vi "PDE_Cal Coef Mtrx.vi"(8 "length":i32, 9 "ks":dbl, 10 "end type":T1 items=["Dirichlet", "Neumann"], 11 "start type":T1 items=["Dirichlet", "Neumann"]) -> (0 "error":i32, 2 "LU of A":T2, 3 "A":T4)   [LabVIEW 2020, in "NI_PDE.lvlib"]
uses:
  <vilib>/gmath/NI_PDE.lvlib
  <vilib>/gmath/pde.llb/Common/PDE_BC Type.ctl
  <vilib>/Analysis/Matrix/Datatypes/RealMatrix.ctl
  <vilib>/Analysis/NI_AALPro.lvlib
  <vilib>/Analysis/Matrix/NI_Matrix.lvlib
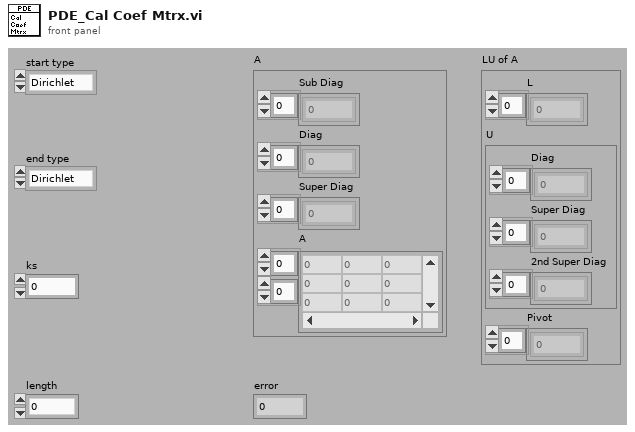
[diagram p1: front panel]
types:
  T1 = typedef "NI_PDE.lvlib/PDE_BC Type.ctl" = i32
  T2 = cluster{"L":dbl[], "U":cluster{"Diag":dbl[], "Super Diag":dbl[], "2nd Super Diag":dbl[]}, "Pivot":i32[]}
  T3 = typedef "NI_Matrix.lvlib/RealMatrix.ctl" = dbl[][]
  T4 = cluster{"Sub Diag":dbl[], "Diag":dbl[], "Super Diag":dbl[], "A":T3}
  T5 = cluster{"Diagonal":dbl[], "Super Diagonal":dbl[], "2nd Super Diagonal":dbl[]}
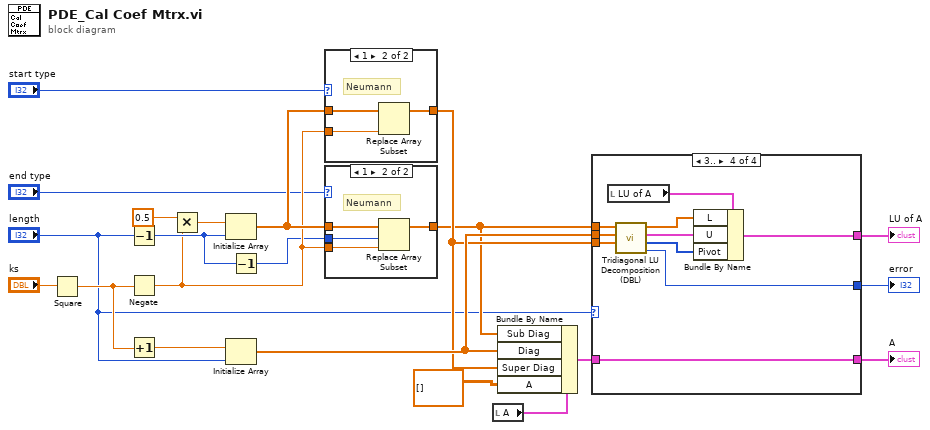
[diagram p0: block diagram]
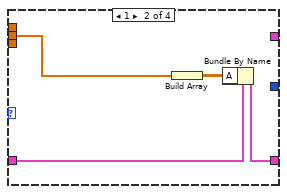
[diagram p3: hidden frame]
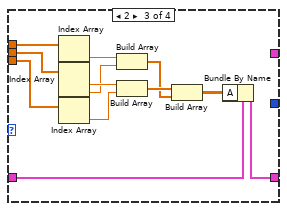
[diagram p4: hidden frame]
diagram:
  n1 = Square(x="ks") -> (x^2=w8:dbl)
  n2 = Decrement(x="length") -> (x-1=w17:i32)
  n3 = Negate(x=w8) -> (-x=w11:dbl)
  n4 = Increment(x=w8) -> (x+1=w21:dbl)
  n5 = Multiply(x=0.5 ("y"), y=w11) -> (x*y=w20:dbl)
  n6 = Initialize Array(w20, w17) -> (w12:dbl[])
  n7 = Initialize Array(w21, "length") -> (w16:dbl[])
  n8 = Decrement(x=w17) -> (x-1=w10:i32)
  n9 = case shown="1" "start type" {
    tunnel: w11 -> [_ w23]
    tunnel: w12 -> [w22 w25]
    tunnel: [w22 w24] -> w13
    frame 0, Default {
      # "Dirichlet"
    }
    frame 1 {
      # "Neumann"
      n10 = Replace Array Subset(array=w25, new element=w23) -> (w24:dbl[])  [unwired: 1 in]
    }
  }
  n11 = case shown="1" "end type" {
    tunnel: w11 -> [_ w28]
    tunnel: w12 -> [w26 w30]
    tunnel: [w26 w29] -> w9
    tunnel: w10 -> [_ w27]
    frame 0, Default {
      # "Dirichlet"
    }
    frame 1 {
      # "Neumann"
      n12 = Replace Array Subset(array=w30, new element=w28, index=w27) -> (w29:dbl[])
    }
  }
  n13 = local read "A"() -> (w7:T4)
  n14 = Bundle By Name(cluster=w7, "Sub Diag"=w9, "Diag"=w16, "Super Diag"=w13, "A"=T3 []) -> (w6:T4)
  n15 = case shown="3.." "length" {
    tunnel: w16 -> [_ w32 w45 w57]
    tunnel: [_ _ _ w56] -> w15
    tunnel: [_ _ _ w55] -> w14
    tunnel: w13 -> [_ _ w43 w54]
    tunnel: w9 -> [_ _ w44 w53]
    tunnel: w6 -> [w31 w35 w47 w48]
    tunnel: [w31 w34 w46 w48] -> w5
    frame 0, Default {
    }
    frame 1 {
      n16 = Build Array(w32) -> (w33:dbl[][])
      n17 = Bundle By Name(cluster=w35, "A"=w33) -> (w34:T4)
    }
    frame 2 {
      n18 = Index Array(array=w44) -> (element=w40:dbl)  [unwired: 1 in]
      n19 = Index Array(array=w45) -> (element #1=w42:dbl, element #2=w39:dbl)  [unwired: 2 in]
      n20 = Index Array(array=w43) -> (element=w41:dbl)  [unwired: 1 in]
      n21 = Build Array(w40, w39) -> (w37:dbl[])
      n22 = Build Array(w42, w41) -> (w38:dbl[])
      n23 = Build Array(w38, w37) -> (w36:dbl[][])
      n24 = Bundle By Name(cluster=w47, "A"=w36) -> (w46:T4)
    }
    frame 3.. {
      n25 = local read "LU of A"() -> (w52:T2)
      n26 = call <vilib>:"Tridiagonal LU Decomposition (DBL).vi"("Super Diagonal"=w54, "Diagonal"=w57, "Sub Diagonal"=w53) -> ("error"=w56:i32, "Pivot"=w49:i32[], "U"=w50:T5, "L"=w51:dbl[])  [unwired: 5 out]
      n27 = Bundle By Name(cluster=w52, "L"=w51, "U"=w50, "Pivot"=w49) -> (w55:T2)
    }
  }
  "LU of A" <- w14
  "error" <- w15
  "A" <- w5
